vi "Delete Buffer.vi"(0 "camHandle IN":u32, 7 "buffHandle IN":u32, 11 "Error IN":errorcluster) -> (15 "Error OUT":errorcluster)   [LabVIEW 2020]
uses:
  Desktop/Vision Point LabVIEW/KYFGLib_lv.lvlib
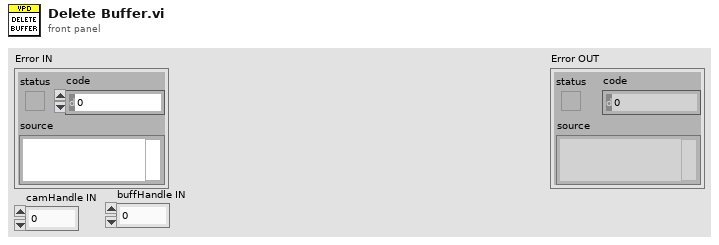
[diagram p1: front panel]
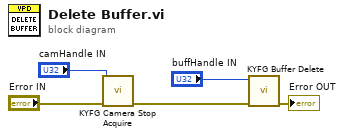
[diagram p0: block diagram]
diagram:
  n1 = call "KYFG Camera Stop Acquire.vi"("error in (no error)"="Error IN", "camHandle"="camHandle IN") -> ("error out"=w5:errorcluster)  [unwired: 8 in, 1 out]
  n2 = call "KYFG Buffer Delete.vi"("error in (no error)"=w5, "streamHandle"="buffHandle IN") -> ("error out"=→"Error OUT":errorcluster)  [unwired: 9 in]
